vi "niUSRP EX Full Duplex (Single Device, Multi Channel)-20221208.vi"() -> ()   [LabVIEW 2021]
doc: "Continuously acquires and generates two communications signals in a synchronous manner using both channels on a two channel device."
uses:
  <instrlib>/niUSRP/niUSRP Timestamp.ctl
  <vilib>/Analysis/3filter.llb/Filter Passband Type.ctl
  <vilib>/addons/Modulation/Analog/controls/Complex Data Waveform.ctl
  <instrlib>/niUSRP/niUSRP Configure Time Start Trigger.vi
  <vilib>/Analysis/3filter.llb/Butterworth Filter (CDB).vi
  <vilib>/addons/Modulation/Analog/MT Upconvert Baseband (Complex).vi
  <instrlib>/niUSRP/niUSRP Fetch Rx Data (2D CDB).vi
  <vilib>/measure/maspectr.llb/FFT Power Spectrum for 1 Chan (CDB).vi
  <instrlib>/niUSRP/niUSRP Write Tx Data (2D CDB).vi
  <vilib>/measure/NI_MABase.lvlib
  <vilib>/measure/NI_MAPro.lvlib
  <vilib>/Analysis/NI_AALBase.lvlib
  <vilib>/addons/Modulation/niAMT.lvlib
panel:
  in  "channel 0 carrier\n frequency [Hz]":dbl=2000000000.0 format="%#_6p"
  in  "channel 1 carrier\n frequency [Hz]":dbl=2000000000.0 format="%#_6p"
  in  "DSP":enum32{"Low Pass Filter", "Modulate"}(tab)
  in  "low cutoff freq (MHz)":dbl(slide)=2.102803738317757 scale=0.0..50.0
  out "x*y":dbl format="%^#.3g"
  in  "carrier frequency (Hz)":dbl=1000.0 min=-0.5 max=0.5 format="%.2f"
  in  "reset? (F)":bool caption="reset?"
  out "Data to Transmit":cdb[][](array[numeric])
  out "IQ Graph 2":dbl[][](graph)
  out "Model":string
  out "error out":errorcluster
  in  "Start Trigger Time":T1={"whole seconds"=1, "fractional seconds"=0.0}
  in  "Tx Active Antenna":string="TX1"
  in  "Tab Control":T2(tab)
  out "IQ Graph":dbl[][](graph)
  out "Baseband Power Spectrum":cluster{"f0":dbl, "df":dbl, "magnitude":dbl[]}[](graph)
  in  "Stop":bool
  in  "Channel 0\nTone Amplitude":dbl=0.707 step=0.05 format="%#.6g"
  in  "Channel 0 \nTone Frequency":dbl=10000.0 format="%#_6p"
  out "Tx Waveform Graph":waveform(dbl)[](graph)
  in  "Waveform Size":dbl=10000.0
  in  "Rx Active Antenna":string="RX2"
  in  "Device Name":refnum<k15>="X310"
  in  "Tx Gain":dbl=1.0 format="%#_6f"
  in  "Tx IQ Rate":dbl=1000000.0 format="%#_6p"
  in  "Rx Gain":dbl=1.0 format="%#_6f"
  in  "Rx IQ Rate":dbl=1000000.0 format="%#_6p"
  # "Rx Settings"
  # "Tx Settings"
  # "For X410 use TX/RX0"
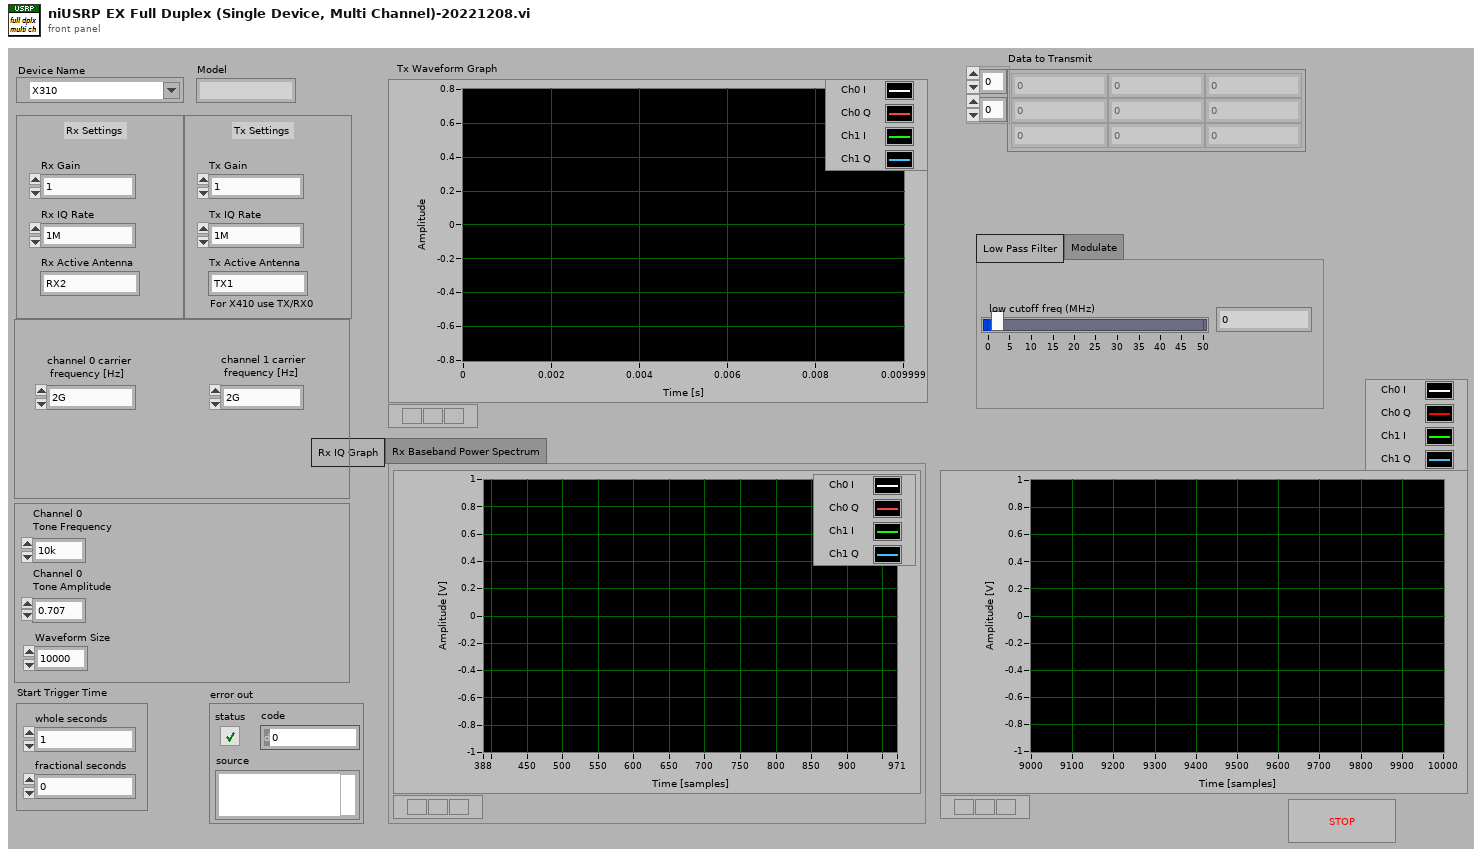
[diagram p1: front panel]
types:
  T1 = typedef "niUSRP Timestamp.ctl" = cluster{"whole seconds":u64, "fractional seconds":dbl}
  T2 = enum32{"Rx IQ Graph", "Rx Baseband Power Spectrum"}
  T3 = typedef "NI_AALBase.lvlib/Filter Passband Type.ctl" = enum32{"Lowpass", "Highpass", "Bandpass", "Bandstop"}
  T4 = typedef "niAMT.lvlib/Complex Data Waveform.ctl" = cluster{"t0":dbl, "dt":dbl, "Y":cdb[]}
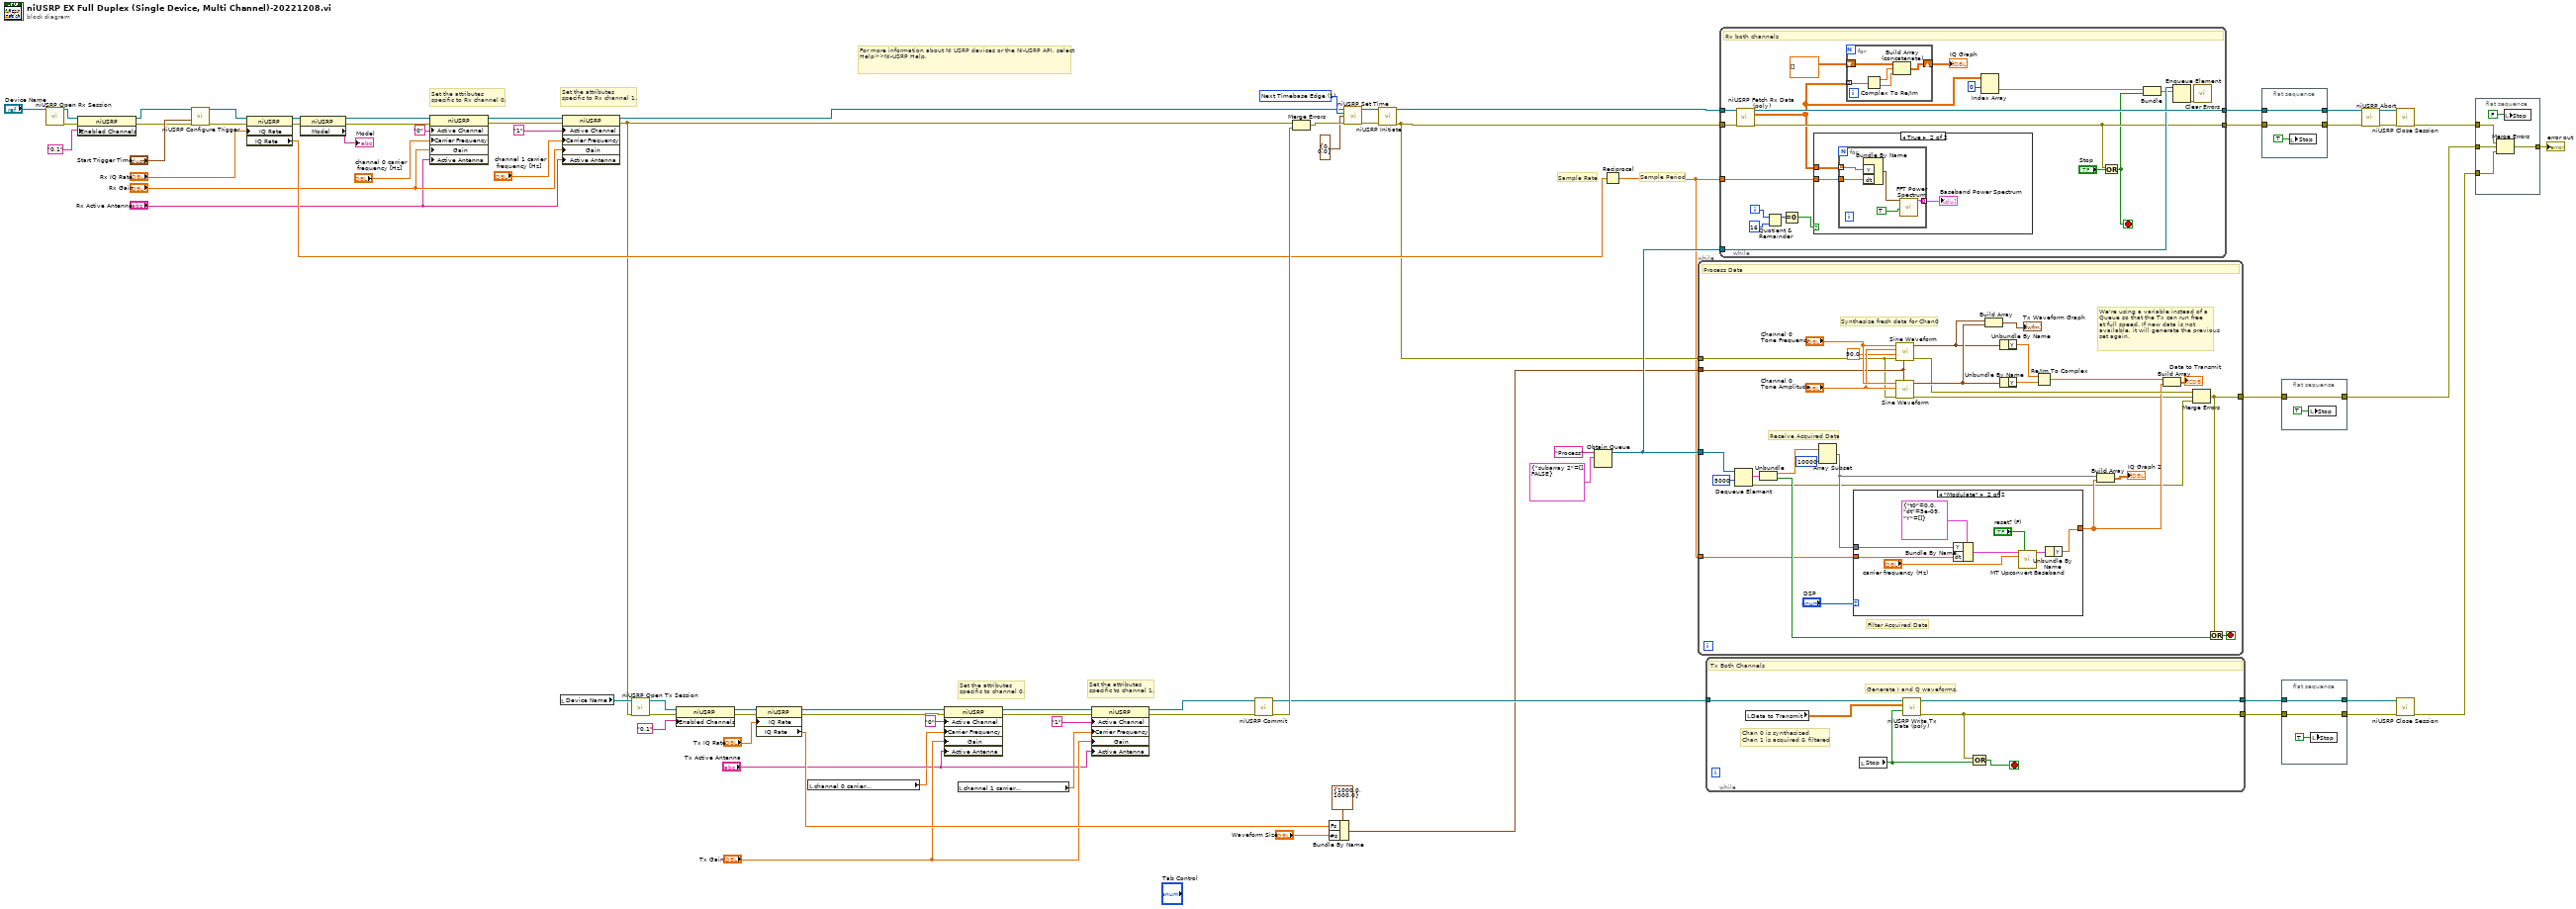
[diagram p0: block diagram]
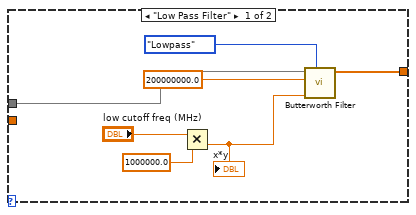
[diagram p2: hidden frame]
diagram:
  w61 = 1 items=["Now", "Next Timebase Edge"] ("apply timestamp")
  # "Set the attributes \nspecific to channel 1."
  # "Set the attributes \nspecific to channel 0."
  # "Set the attributes \nspecific to Rx channel 1."
  # "Set the attributes \nspecific to Rx channel 0."
  # "Sample Rate"
  # "Sample Period"
  # "For more information about NI USRP devices or the NI-USRP API, select Help>>NI-USRP Help."
  n1 = call <instrlib>:"niUSRP Open Rx Session.vi"("device names"="Device Name") -> ("session handle out"=w60:refnum<k15>, "error out"=w59:errorcluster)  [unwired: 13 in]
  n2 = property class="niUSRP"(reference=w60, error in=w59, "Enabled Channels"="0,1" ("Configuration:Enabled Channels")) -> (reference out=w58:refnum<k15>, error out=w57:errorcluster)
  n3 = call-poly <instrlib>:"niUSRP Configure Trigger.vi"("session handle"=w58, "start trigger time"="Start Trigger Time", "error in (no error)"=w57) -> ("session handle out"=w54:refnum<k15>, "error out"=w53:errorcluster)  [unwired: 11 in]
  n4 = property class="niUSRP"(reference=w54, error in=w53, "IQ Rate"="Rx IQ Rate") -> (reference out=w49:refnum<k15>, error out=w50:errorcluster, "IQ Rate"=w51:dbl)
  n5 = property class="niUSRP"(reference=w49, error in=w50) -> (reference out=w46:refnum<k15>, error out=w3:errorcluster, "Model"=→"Model":string)
  n6 = property class="niUSRP"(reference=w46, error in=w3, "Active Channel"="0", "Carrier Frequency"="channel 0 carrier\n frequency [Hz]", "Gain"="Rx Gain", "Active Antenna"="Rx Active Antenna") -> (reference out=w22:refnum<k15>, error out=w21:errorcluster)
  n7 = local read "Device Name"() -> (w71:refnum<k15>)
  n8 = property class="niUSRP"(reference=w22, error in=w21, "Active Channel"="1", "Carrier Frequency"="channel 1 carrier\n frequency [Hz]", "Gain"="Rx Gain", "Active Antenna"="Rx Active Antenna") -> (reference out=w48:refnum<k15>, error out=w47:errorcluster)
  n9 = call <instrlib>:"niUSRP Open Tx Session.vi"("device names"=w71, "error in (no error)"=w47) -> ("session handle out"=w56:refnum<k15>, "error out"=w55:errorcluster)  [unwired: 12 in]
  n10 = property class="niUSRP"(reference=w56, error in=w55, "Enabled Channels"="0,1" ("Configuration:Enabled Channels")) -> (reference out=w43:refnum<k15>, error out=w42:errorcluster)
  n11 = property class="niUSRP"(reference=w43, error in=w42, "IQ Rate"="Tx IQ Rate") -> (reference out=w39:refnum<k15>, error out=w40:errorcluster, "IQ Rate"=w38:dbl)
  n12 = local read "channel 0 carrier\n frequency [Hz]"() -> (w11:dbl)
  n13 = property class="niUSRP"(reference=w39, error in=w40, "Active Channel"="0", "Carrier Frequency"=w11, "Gain"="Tx Gain", "Active Antenna"="Tx Active Antenna") -> (reference out=w15:refnum<k15>, error out=w14:errorcluster)
  n14 = local read "channel 1 carrier\n frequency [Hz]"() -> (w10:dbl)
  n15 = property class="niUSRP"(reference=w15, error in=w14, "Active Channel"="1", "Carrier Frequency"=w10, "Gain"="Tx Gain", "Active Antenna"="Tx Active Antenna") -> (reference out=w36:refnum<k15>, error out=w37:errorcluster)
  n16 = call <instrlib>:"niUSRP Commit.vi"("session handle"=w36, "error in (no error)"=w37) -> ("session handle out"=w73:refnum<k15>, "error out"=w74:errorcluster)  [unwired: 12 in]
  n17 = Merge Errors(w47, w74) -> (w63:errorcluster)
  n18 = Bundle By Name(cluster=cluster{"Fs":dbl, "#s":dbl} {"Fs"=1000.0, "#s"=1000.0} ("sampling info"), "Fs"=w38, "#s"="Waveform Size") -> (w6:cluster{"Fs":dbl, "#s":dbl})
  n19 = call <instrlib>:"niUSRP Set Time.vi"("session handle"=w48, "apply timestamp"=w61, "timestamp"=T1 {"whole seconds"=0, "fractional seconds"=0.0}, "error in (no error)"=w63) -> ("session handle out"=w65:refnum<k15>, "error out"=w64:errorcluster)  [unwired: 10 in]
  n20 = call <instrlib>:"niUSRP Initiate.vi"("session handle"=w65, "error in (no error)"=w64) -> ("session handle out"=w77:refnum<k15>, "error out"=w5:errorcluster)  [unwired: 12 in]
  n21 = Obtain Queue(name (unnamed)="Process", element data type=cluster{"subarray 2":cdb[], bool} {"subarray 2"=[], FALSE}) -> (queue out=w8:refnum<queue>)  [unwired: 3 in, 2 out]
  n22 = Reciprocal(x=w51) -> (1/x=w4:dbl)
  n23 = while {
    tunnel: w8 -> [w105]
    tunnel: [w79] -> w1
    tunnel: w6 -> [w90]
    tunnel: w5 -> [w86]
    tunnel: w4 -> [w81]
    stop <- w80 stop-if-true
    # "We're using a variable instead of a \nQueue so that the Tx can run free\nat full speed. If new data is not\navailable, it will generate the previous\nset again."
    # "Filter Acquired Data"
    # "Synthesize fresh data for Chan0"
    # "Receive Acquired Data"
    # "Process Data"
    n24 = Dequeue Element(queue=w105, timeout in ms (-1)=5000) -> (element=w104:cluster{"subarray 2":cdb[], bool}, error out=w85:errorcluster)  [unwired: 1 in, 2 out]
    n25 = Unbundle(w104) -> ("subarray 2"=w102:cdb[], w103:bool)
    n26 = Array Subset(array=w102, length=10000) -> (w100:cdb[])  [unwired: 1 in]
    n27 = case shown="\"Modulate\"" "DSP" {
      tunnel: w100 -> [w109 w118]
      tunnel: [w108 w115] -> w88
      tunnel: w81 -> [_ w113]
      frame "Low Pass Filter" {
        n28 = Multiply(x="low cutoff freq (MHz)", y=1000000.0 ("x")) -> (x*y=w107:dbl)
        "x*y" <- w107
        n29 = call-poly <vilib>:"Butterworth Filter.vi"("filter type"=Filter_Passband_Type."Lowpass", "low cutoff freq: fl"=w107, "sampling freq: fs"=200000000.0, "X"=w109) -> ("Filtered X"=w108:cdb[])  [unwired: 4 in, 1 out]
      }
      frame "Modulate" {
        n30 = Bundle By Name(cluster=T4 {"t0"=0.0, "dt"=5e-09, "Y"=[]} ("baseband waveform (complex)"), "Y"=w118, "dt"=w113) -> (w119:T4)
        n31 = call-poly <vilib>:"MT Upconvert Baseband.vi"("complex waveform"=w119, "reset? (F)"="reset? (F)", "carrier frequency (Hz)"="carrier frequency (Hz)") -> ("upconverted waveform (complex)"=w116:T4)  [unwired: 11 in, 1 out]
        n32 = Unbundle By Name(w116) -> ("Y"=w115:cdb[])
      }
    }
    n33 = call <vilib>:"Sine Waveform.vi"("sampling info"=w90, "error in (no error)"=w86, "phase"=90.0, "amplitude"="Channel 0\nTone Amplitude", "frequency"="Channel 0 \nTone Frequency") -> ("error out"=w91:errorcluster, "signal out"=w96:waveform(dbl))  [unwired: 5 in]
    n34 = call <vilib>:"Sine Waveform.vi"("sampling info"=w90, "error in (no error)"=w86, "amplitude"="Channel 0\nTone Amplitude", "frequency"="Channel 0 \nTone Frequency") -> ("error out"=w87:errorcluster, "signal out"=w97:waveform(dbl))  [unwired: 6 in]
    n35 = Build Array(w96, w97) -> (→"Tx Waveform Graph":waveform(dbl)[])
    n36 = Unbundle By Name(w96) -> ("Y"=w95:dbl[])
    n37 = Unbundle By Name(w97) -> ("Y"=w94:dbl[])
    n38 = Re/Im To Complex(1:w94, 2:w95) -> (0:w83:cdb[])
    n39 = Build Array(w100, w88) -> (→"IQ Graph 2":cdb[][])
    n40 = Build Array(w83, w88) -> (→"Data to Transmit":cdb[][])
    n41 = Merge Errors(w91, w87, w85) -> (w79:errorcluster)
    n42 = Or(x=w79, y=w103) -> (x .or. y?=w80:bool)
  }
  n43 = while {
    tunnel: w73 -> [w126]
    tunnel: [w125] -> w34
    tunnel: [w123] -> w27
    stop <- w124 stop-if-true
    # "Chan 0 is synthesized\nChan 1 is acquired & filtered"
    # "Generate I and Q waveforms."
    # "Tx Both Channels"
    n44 = local read "Data to Transmit"() -> (w121:cdb[][])
    n45 = local read "Stop"() -> (w122:bool)
    n46 = call-poly <instrlib>:"niUSRP Write Tx Data (poly).vi"("session handle"=w126, "data"=w121, "end of data?"=w122) -> ("session handle out"=w123:refnum<k15>, "error out"=w125:errorcluster)  [unwired: 11 in]
    n47 = Compound Arithmetic op=OR(w125, w122) -> (w124:bool)
  }
  n48 = while {
    tunnel: w77 -> [w145]
    tunnel: w5 -> [w144]
    tunnel: [w130] -> w32
    tunnel: [w143] -> w29
    tunnel: w4 -> [w137]
    tunnel: w8 -> [w135]
    i -> [w140]
    stop <- w129 stop-if-true
    # "Rx both channels"
    n49 = call-poly <instrlib>:"niUSRP Fetch Rx Data (poly).vi"("session handle"=w145, "error in (no error)"=w144) -> ("session handle out"=w143:refnum<k15>, "data"=w127:cdb[][], "error out"=w130:errorcluster)  [unwired: 10 in, 1 out]
    n50 = Quotient & Remainder(x=w140, y=16) -> (x-y*floor(x/y)=w142:i32)  [unwired: 1 out]
    n51 = Equal To 0?(x=w142) -> (x = 0?=w139:bool)
    n52 = case shown="True" w139 {
      tunnel: w127 -> [_ w153]
      tunnel: w137 -> [_ w152]
      frame False {
      }
      frame True {
        n53 = for {
          tunnel: w153 -> [w156] mode=indexing
          tunnel: w152 -> [w155]
          tunnel: [w154] -> w151 mode=indexing
          n54 = Bundle By Name("Y"=w156, "dt"=w155) -> (w157:waveform(cdb))  [unwired: 1 in]
          n55 = call-poly <vilib>:"FFT Power Spectrum.vi"("dB On (F)"=TRUE, "time signal"=w157) -> ("power spectrum"=w154:cluster{"f0":dbl, "df":dbl, "magnitude":dbl[]})  [unwired: 6 in, 3 out]
        }
        "Baseband Power Spectrum" <- w151
      }
    }
    n56 = for {
      tunnel: w127 -> [w146] mode=indexing
      shift-right: [w148] -> w136
      shift-left: dbl[][] [] -> [w147]
      n57 = Complex To Re/Im(x + iy=w146) -> (x=w150:dbl[], y=w149:dbl[])
      n58 = Build Array (concatenate)(w147, w150, w149) -> (w148:dbl[][])
    }
    "IQ Graph" <- w136
    n59 = Index Array(array=w127, index (row)=0) -> (element=w133:cdb[])  [unwired: 1 in]
    n60 = Or(x=w130, y="Stop") -> (x .or. y?=w129:bool)
    n61 = Bundle("data"=w133, w129) -> (w132:cluster{"data":cdb[], bool})  [unwired: 1 in]
    n62 = Enqueue Element(queue=w135, element=w132) -> (error out=w134:errorcluster)  [unwired: 2 in, 2 out]
    n63 = call <vilib>:"Clear Errors.vi"("error in (no error)"=w134) -> ()  [unwired: 5 in, 2 out]
  }
  n64 = flat-sequence {
    tunnel: [w160] -> w31
    tunnel: w32 -> [w160]
    tunnel: [w159] -> w30
    tunnel: w29 -> [w159]
    frame #0 {
      n65 = local write "Stop"(TRUE ("STOP")) -> ()
    }
  }
  n66 = flat-sequence {
    tunnel: [w162] -> w2
    tunnel: w1 -> [w162]
    frame #0 {
      n67 = local write "Stop"(TRUE ("STOP")) -> ()
    }
  }
  n68 = flat-sequence {
    tunnel: [w165] -> w33
    tunnel: w34 -> [w165]
    tunnel: [w164] -> w28
    tunnel: w27 -> [w164]
    frame #0 {
      n69 = local write "Stop"(TRUE ("STOP")) -> ()
    }
  }
  n70 = call <instrlib>:"niUSRP Abort.vi"("session handle"=w30, "error in (no error)"=w31) -> ("session handle out"=w70:refnum<k15>, "error out"=w69:errorcluster)  [unwired: 12 in]
  n71 = call <instrlib>:"niUSRP Close Session.vi"("session handle"=w70, "error in (no error)"=w69) -> ("error out"=w26:errorcluster)  [unwired: 13 in]
  n72 = call <instrlib>:"niUSRP Close Session.vi"("session handle"=w28, "error in (no error)"=w33) -> ("error out"=w25:errorcluster)  [unwired: 13 in]
  n73 = flat-sequence {
    tunnel: w26 -> [w170]
    tunnel: w25 -> [w169]
    tunnel: [w168] -> w24
    tunnel: w2 -> [w167]
    frame #0 {
      n74 = Merge Errors(w170, w167, w169) -> (w168:errorcluster)
      n75 = local write "Stop"(FALSE ("STOP")) -> ()
    }
  }
  "error out" <- w24
